vi "Tree.vi"() -> ()   [LabVIEW 2019, in "API.lvclass"]
uses:
  API.lvclass
  Framework/Instrument Types/CBridge/Typedefs/CBridge.Commands--Enum.ctl
  Framework/Instrument Types/Cryostat/Typedefs/Cryostat.commands--enum.ctl
  Framework/Instrument Types/Delay Line/Typedefs/DelayLine.Commands--Enum.ctl
  Framework/Instrument Types/Lockin/Typedefs/LockinAPI.commands--Enum.ctl
  Framework/Instrument Types/Strain/Typedefs/Strain.Commands--Enum.ctl
  Framework/Instrument Types/SCPI/Typedefs/SCPI.Commands--Enum.ctl
  Framework/Instrument Types/VNA/Typedefs/VNA.Commands--Enum.ctl
  Framework/Instrument Types/SignalGenerator/Typedefs/SignalGenerator.Commands--Enum.ctl
  b0305475-a326-4e49-ab7e-c40734a1c22e.vi
  <vilib>/Utility/Data Type/Get Numeric Information.vi
  Framework/Instrument Types/CBridge/Instrument.CBridge.lvclass
  Framework/Instrument Types/Cryostat/Instrument.Cryostat.lvclass
  Framework/Instrument Types/Delay Line/Instrument.DelayLine.lvclass
  Framework/Instrument Types/Lockin/Instrument.LockinAPI.lvclass
  Framework/Instrument Types/Strain/Instrument.Strain.lvclass
  Framework/Instrument Types/SCPI/Instrument.SCPI.lvclass
  Framework/Instrument Types/VNA/Instrument.VNA.lvclass
  Framework/Instrument Types/SignalGenerator/Instrument.SignalGenerator.lvclass
  <vilib>/Utility/Data Type/NI_Data Type.lvlib
panel:
  out "delimited string":string
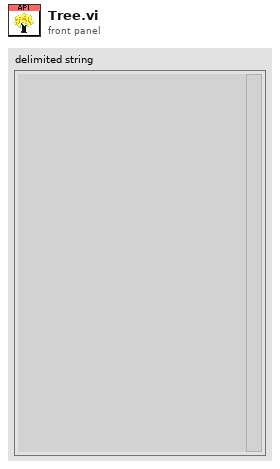
[diagram p1: front panel]
types:
  T1 = typedef "Instrument.SignalGenerator.lvclass/SignalGenerator.Commands--Enum.ctl" = enum16{"setFrequency", "setFunction", "setLevel", "setOffset", "setPhase", "setPower"}
  T2 = typedef "Instrument.VNA.lvclass/VNA.Commands--Enum.ctl" = enum16{"getData", "setAverage", "setFormat", "setMeasurement", "setPower", "setSweep"}
  T3 = typedef "Instrument.SCPI.lvclass/SCPI.Commands--Enum.ctl" = enum16{"sendSCPI", "receiveSCPI"}
  T4 = typedef "Instrument.Strain.lvclass/Strain.Commands--Enum.ctl" = enum16{"getStrain", "setStrain"}
  T5 = typedef "Instrument.LockinAPI.lvclass/LockinAPI.commands--Enum.ctl" = enum16{"setAI", "setAO", "setAO_Amplitude", "setAO_DC", "setAO_Frequency", "setAO_Phase", "setAO_Function", "setAO_I+", "setREF", "setREF_Frequency", "setREF_Phase", "setREF_TC", "setREF_Roll-Off", "setDAQ", "setSampling", "setOffset", "setState", "getState", "getAO", "getAI", "getResults", "getSampling", "getAOconfig", "getREFconfig", "setInputGain", "setOutputGain", "getInputGain", "getOutputGain", "setSamplingMode", "getSamplingMode", "setSweep", "setSweepTime", "setSweepTable", "getStatus", "getSweepResults", "getSweepWaveforms", "startSweep", "stopSweep", "setAUX", "getAUX"}
  T6 = typedef "Instrument.DelayLine.lvclass/DelayLine.Commands--Enum.ctl" = enum16{"getDelay", "setDelay"}
  T7 = typedef "Instrument.Cryostat.lvclass/Cryostat.commands--enum.ctl" = enum16{"getLN2Level", "getLHeLevel", "getMagnet", "getMagnetVector", "setMagnet", "setMagnetVector", "getAngle", "setAngle", "getTemperature", "setTemperature", "getHeater", "setHeater", "getChamber", "setChamber", "getPressure"}
  T8 = typedef "Instrument.CBridge.lvclass/CBridge.Commands--Enum.ctl" = enum16{"getCapacitance"}
  T9 = typedef "NI_Data Type.lvlib/Type Definition Info.ctl" = cluster{"Name":string, "Timestamp":u32}
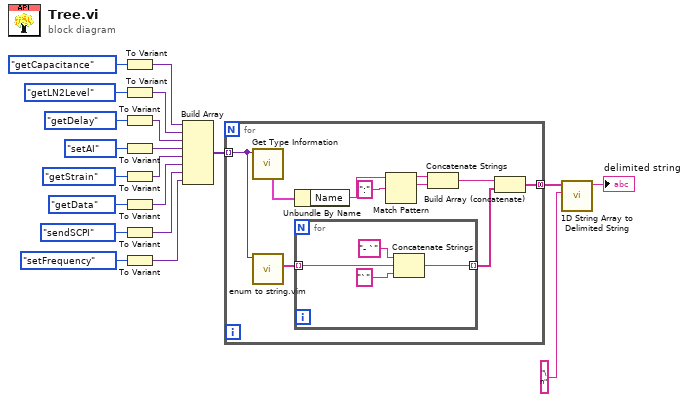
[diagram p0: block diagram]
diagram:
  n1 = To Variant(anything=CBridge.Commands--Enum."getCapacitance" ("Commands")) -> (Variant=w13:variant)
  n2 = To Variant(anything=Cryostat.commands--enum."getLN2Level" ("commands")) -> (Variant=w12:variant)
  n3 = To Variant(anything=DelayLine.Commands--Enum."getDelay" ("command")) -> (Variant=w11:variant)
  n4 = To Variant(anything=LockinAPI.commands--Enum."setAI" ("commands")) -> (Variant=w10:variant)
  n5 = To Variant(anything=Strain.Commands--Enum."getStrain" ("Command")) -> (Variant=w9:variant)
  n6 = To Variant(anything=VNA.Commands--Enum."getData" ("Commands")) -> (Variant=w8:variant)
  n7 = To Variant(anything=SCPI.Commands--Enum."sendSCPI" ("Commands")) -> (Variant=w7:variant)
  n8 = To Variant(anything=SignalGenerator.Commands--Enum."setFrequency" ("Commands")) -> (Variant=w6:variant)
  n9 = Build Array(w13, w12, w11, w10, w9, w8, w7, w6) -> (w5:variant[])
  n10 = for {
    tunnel: w5 -> [w30] mode=indexing
    tunnel: [w28] -> w1 mode=concatenating
    n11 = call <vilib>:"Get Type Information.vi"("variant"=w30) -> ("type definition info"=w29:T9)  [unwired: 6 in, 4 out]
    n12 = call "enum to string.vim"("enum in"=w30) -> ("strings out"=w27:string[])  [unwired: 9 in, 1 out]
    n13 = Unbundle By Name(w29) -> ("Name"=w25:string)
    n14 = for {
      tunnel: w27 -> [w34] mode=indexing
      tunnel: [w31] -> w26 mode=indexing
      n15 = Concatenate Strings("- `" ("string"), w34, "`" ("string")) -> (w31:string)
    }
    n16 = Match Pattern(string=w25, regular expression=":" ("replace string (\"\")")) -> (before substring=w23:string, match substring=w22:string)  [unwired: 1 in, 2 out]
    n17 = Concatenate Strings(w23, w22) -> (w21:string)
    n18 = Build Array (concatenate)(w21, w26) -> (w28:string[])
  }
  n19 = call <vilib>:"1D String Array to Delimited String.vi"("delimiter"="\n", "string array"=w1) -> ("delimited string"=→"delimited string":string)  [unwired: 9 in]
